vi "Teleop.vi"(10 "Match Info":T1={"Autonomous Elapsed Seconds"=0.0, "TeleOp Elapsed Seconds"=0.0, "Disabled Elapsed Seconds"=0.0, "Visited Autonomous"=FALSE, "Visited TeleOp"=FALSE, "Visited Disabled"=FALSE, "Autonomous Settings"={"Autonomous Style"=enum."Independent", "VI Refnum"=refnum}}, 11 "Call Context":T2) -> ()   [LabVIEW 2019]
doc: "This VI is called for each TeleOp packet received from the DS where the robot is not disabled. It is often used to read from the joysticks and update I/O or to update setpoints for timed control loops. It should complete and return within 20 milliseconds or it may miss DS packets."
uses:
  <vilib>/Rock Robotics/WPI/DriverStation/WPI_DriverStationDerivedRobotMode.ctl
  <vilib>/Rock Robotics/WPI/DriverStation/WPI_DriverStationMatch Info.ctl
  <vilib>/Rock Robotics/WPI/Utilities/WPI_GetSetVariantRefNum.vi
  <vilib>/Rock Robotics/Network Tables/NT Write Boolean Array.vi
  <vilib>/Rock Robotics/Network Tables/NT Write Numeric Array.vi
  <vilib>/Rock Robotics/Network Tables/NT Read Boolean.vi
  <vilib>/Rock Robotics/Network Tables/NT Read Number.vi
panel:
  out "Sample Slider 0":dbl(slide) scale=0.0..5.0
  out "Sample Boolean 1":bool
  out "Sample Boolean 0":bool
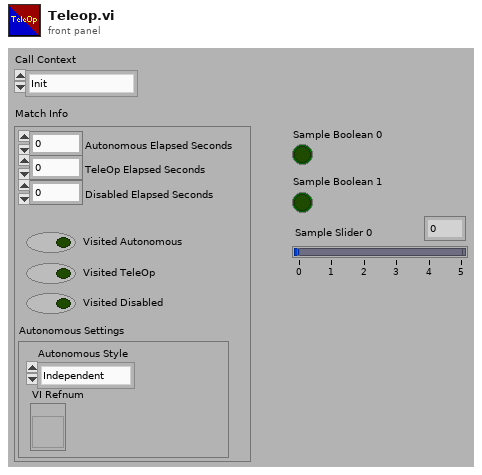
[diagram p1: front panel]
types:
  T1 = typedef "WPI_DriverStationMatch Info.ctl" = cluster{"Autonomous Elapsed Seconds":dbl, "TeleOp Elapsed Seconds":dbl, "Disabled Elapsed Seconds":dbl, "Visited Autonomous":bool, "Visited TeleOp":bool, "Visited Disabled":bool, "Autonomous Settings":cluster{"Autonomous Style":enum16{"Iterative", "Independent"}, "VI Refnum":refnum<vi>}}
  T2 = typedef "WPI_DriverStationDerivedRobotMode.ctl" = enum16{"Init", "Execute", "Stop"}
  T3 = typedef "WPI_RobotDriveDevRef.ctl" = cluster{"DevStatus":errorcluster, "Motors[]":T4[], "Square Inputs":bool, "Max Output":dbl}
  T4 = typedef "WPI_MotorControlDeviceRef.ctl" = cluster{"DeviceStatus":errorcluster, "Type":T5, "PWM":cluster{"PWM Channel":T6, "DeadBand":T7}, "CAN":cluster{"Device Number":u8, "SetOutput VI Ref":variant, "GetOutput VI Ref":variant, "Enable VI Ref":variant, "Disable VI Ref":variant, "Data":variant}, "Invert":bool, "DIO PWM":cluster{"PWM \"Enable\" Channel":T6, "DIOChannel":T8, "PWM Rate":dbl}}
  T5 = typedef "WPI_MotorControlType.ctl" = enum16{"PWM", "CAN", "DIO PWM"}
  T6 = typedef "FPGA_DIOPWMChannel.ctl" = enum8{"PWM 0", "PWM 1", "PWM 2", "PWM 3", "PWM 4", "PWM 5", "PWM 6", "PWM 7", "PWM 8", "PWM 9", "PWM MXP 0", "PWM MXP 1", "PWM MXP 2", "PWM MXP 3", "PWM MXP 4", "PWM MXP 5", "PWM MXP 6", "PWM MXP 7", "PWM MXP 8", "PWM MXP 9", "Invalid"}
  T7 = typedef "WPI_PWMDeadband.ctl" = cluster{"Name":string, "maxPositivePwm":i32, "minPositivePwm":i32, "centerPwm":i32, "maxNegativePwm":i32, "minNegativePwm":i32, "angularRange":u16}
  T8 = typedef "FPGA_DIOChannel.ctl" = enum8{"DIO 0", "DIO 1", "DIO 2", "DIO 3", "DIO 4", "DIO 5", "DIO 6", "DIO 7", "DIO 8", "DIO 9", "DIO MXP 0", "DIO MXP 1", "DIO MXP 2", "DIO MXP 3", "DIO MXP 4", "DIO MXP 5", "DIO MXP 6", "DIO MXP 7", "DIO MXP 8", "DIO MXP 9", "DIO MXP 10", "DIO MXP 11", "DIO MXP 12", "DIO MXP 13", "DIO MXP 14", "DIO MXP 15", "SPI Port CS1", "SPI Port CS2", "SPI Port CS3", "SPI Port MISO", "SPI Port MOSI", "Invalid"}
  T9 = typedef "WPI_JoystickDevRef.ctl" = cluster{"Device":T10}
  T10 = typedef "WPI_JoystickDeviceEnum.ctl" = enum16{"USB 0", "USB 1", "USB 2", "USB 3", "USB 4", "USB 5"}
  T11 = typedef "WPI_DigitalOutputDevRef.ctl" = cluster{"DIO Channel":T8, "DevStatus":errorcluster}
  T12 = typedef "WPI_AnalogChannelDevRef.ctl" = cluster{"DevStatus":errorcluster, "Analog Channel":T13}
  T13 = typedef "FPGA_AIChannel.ctl" = enum8{"AI 0", "AI 1", "AI 2", "AI 3", "AI MXP 0", "AI MXP 1", "AI MXP 2", "AI MXP 3", "Invalid"}
  T14 = typedef "WPI_GyroDevRef.ctl" = cluster{"DevStatus":errorcluster, "Analog Channel":T13, "Gain (VoltsPerDegree/Second)":dbl, "Gyro Type":enum16{"Analog", "XRS450"}, "Handle":i32, "SPI Bus":T15, "Device Found":bool, "Sample Rate":dbl, "Calibrate On Open":bool, "Offset":dbl}
  T15 = typedef "spi_bus.ctl" = enum16{"SPI On-Board, CS0", "SPI On-Board, CS1", "SPI On-Board, CS2", "SPI On-Board, CS3", "SPI MXP", "Invalid"}
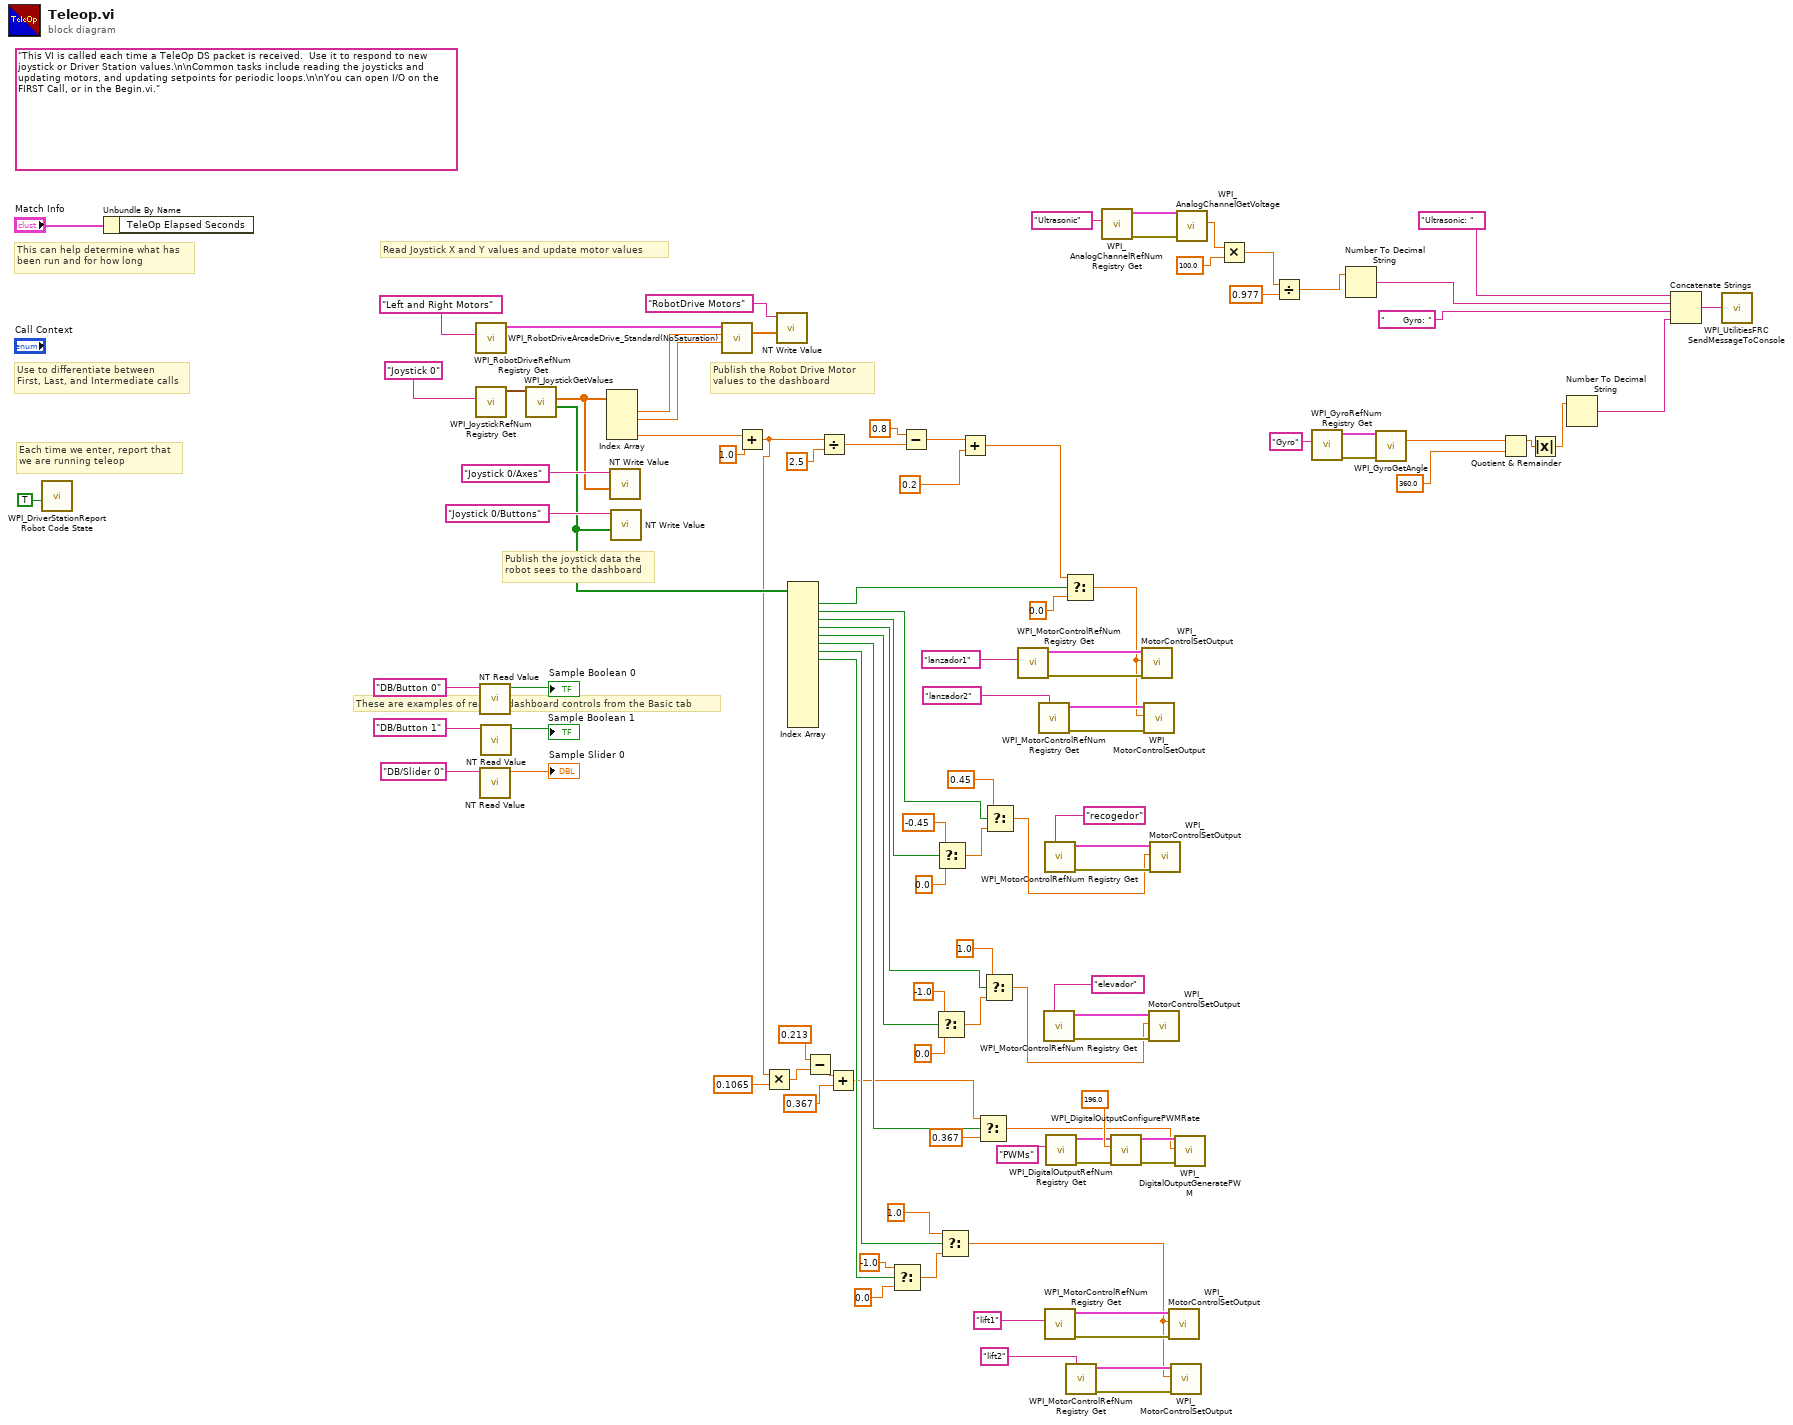
[diagram p0: block diagram]
diagram:
  (unwired) "This VI is called each time a TeleOp DS packet is received.  Use it to respond to new joystick or Driver Station values.\n\nCommon tasks include reading the joysticks and updating motors, and updating setpoints for periodic loops.\n\nYou can open I/O on the FIRST Call, or in the Begin.vi."
  # "These are examples of reading dashboard controls from the Basic tab"
  # "Publish the Robot Drive Motor\nvalues to the dashboard"
  # "Publish the joystick data the\nrobot sees to the dashboard"
  # "Each time we enter, report that\nwe are running teleop"
  # "Use to differentiate between\nFirst, Last, and Intermediate calls"
  # "This can help determine what has\nbeen run and for how long"
  # "Read Joystick X and Y values and update motor values"
  n1 = call <vilib>:"WPI_DriverStationReport Robot Code State.vi"("TeleOp"=TRUE ("Autonomous")) -> ()  [unwired: 10 in, 1 out]
  n2 = Unbundle By Name("Match Info") -> ()  [unwired: 1 out]
  n3 = call <vilib>:"WPI_RobotDriveRefNum Registry Get.vi"("refnum name"="Left and Right Motors") -> ("RobotDriveDevRef"=w103:T3)  [unwired: 1 in, 9 out]
  n4 = call <vilib>:"WPI_JoystickRefNum Registry Get.vi"("refnum name"="Joystick 0") -> ("JoystickDevRef"=w100:T9)  [unwired: 1 in, 9 out]
  n5 = call-poly <vilib>:"NT Read Value.vi"("Name"="DB/Button 0" ("refnum name")) -> ("Boolean"=→"Sample Boolean 0":bool)  [unwired: 9 in, 1 out]
  n6 = call-poly <vilib>:"NT Read Value.vi"("Name"="DB/Slider 0" ("refnum name")) -> ("Numeric"=→"Sample Slider 0":dbl)  [unwired: 9 in, 1 out]
  n7 = call-poly <vilib>:"NT Read Value.vi"("Name"="DB/Button 1" ("refnum name")) -> ("Boolean"=→"Sample Boolean 1":bool)  [unwired: 9 in, 1 out]
  n8 = call <vilib>:"WPI_JoystickGetValues.vi"("JoystickDevRef"=w100) -> ("Buttons"=w86:bool[], "Axes"=w95:dbl[])  [unwired: 6 in, 3 out]
  n9 = Index Array(array=w95) -> (element #1=w102:dbl, element #2=w98:dbl, element #4=w33:dbl)  [unwired: 4 in, 1 out]
  n10 = call-poly <vilib>:"NT Write Value.vi"("Numeric Array"=w95, "Name"="Joystick 0/Axes") -> ()  [unwired: 9 in, 1 out]
  n11 = call-poly <vilib>:"NT Write Value.vi"("Boolean Array"=w86, "Name"="Joystick 0/Buttons") -> ()  [unwired: 9 in, 1 out]
  n12 = call <vilib>:"WPI_RobotDriveArcadeDrive_Standard(NoSaturation).vi"("Y axis value"=w98, "X axis value"=w102, "RobotDriveDevRef"=w103) -> ("Motor Values"=w88:dbl[])  [unwired: 1 in, 7 out]
  n13 = Add(x=w33, y=1.0) -> (x+y=w11:dbl)
  n14 = Multiply(x=w11, y=0.1065) -> (x*y=w9:dbl)
  n15 = call-poly <vilib>:"NT Write Value.vi"("Numeric Array"=w88, "Name"="RobotDrive Motors") -> ()  [unwired: 9 in, 1 out]
  n16 = Index Array(array=w86) -> (element #1=w75:bool, element #2=w59:bool, element #3=w56:bool, element #4=w45:bool, element #5=w44:bool, element #6=w43:bool, element #7=w17:bool, element #8=w16:bool)  [unwired: 16 in, 8 out]
  n17 = Subtract(x=0.213, y=w9) -> (x-y=w7:dbl)
  n18 = Divide(x=w11, y=2.5) -> (x/y=w29:dbl)
  n19 = Add(x=w7, y=0.367) -> (x+y=w5:dbl)
  n20 = Select(t=-1.0, s=w16, f=0.0) -> (s? t:f=w18:dbl)
  n21 = Subtract(x=0.8, y=w29) -> (x-y=w28:dbl)
  n22 = Select(t=-1.0, s=w44, f=0.0 ("t")) -> (s? t:f=w48:dbl)
  n23 = Select(t=-0.45, s=w56, f=0.0 ("t")) -> (s? t:f=w57:dbl)
  n24 = Select(t=1.0, s=w17, f=w18) -> (s? t:f=w12:dbl)
  n25 = Add(x=w28, y=0.2) -> (x+y=w26:dbl)
  n26 = Select(t=w5, s=w43, f=0.367) -> (s? t:f=w13:dbl)
  n27 = Select(t=1.0, s=w45, f=w48) -> (s? t:f=w50:dbl)
  n28 = Select(t=0.45, s=w59, f=w57) -> (s? t:f=w60:dbl)
  n29 = call <vilib>:"WPI_MotorControlRefNum Registry Get.vi"("refnum name"="lanzador1") -> ("error out"=w83:errorcluster, "MotorControlDevRef"=w84:T4)  [unwired: 9 in]
  n30 = call <vilib>:"WPI_MotorControlRefNum Registry Get.vi"("refnum name"="lanzador2") -> ("error out"=w80:errorcluster, "MotorControlDevRef"=w81:T4)  [unwired: 9 in]
  n31 = call <vilib>:"WPI_MotorControlRefNum Registry Get.vi"("refnum name"="elevador") -> ("error out"=w52:errorcluster, "MotorControlDevRef"=w53:T4)  [unwired: 9 in]
  n32 = call <vilib>:"WPI_MotorControlRefNum Registry Get.vi"("refnum name"="recogedor") -> ("error out"=w77:errorcluster, "MotorControlDevRef"=w78:T4)  [unwired: 9 in]
  n33 = call <vilib>:"WPI_MotorControlRefNum Registry Get.vi"("refnum name"="lift1") -> ("error out"=w41:errorcluster, "MotorControlDevRef"=w42:T4)  [unwired: 9 in]
  n34 = call <vilib>:"WPI_DigitalOutputRefNum Registry Get.vi"("refnum name"="PWMs") -> ("error out"=w22:errorcluster, "DigitalOutputDevRef"=w23:T11)  [unwired: 9 in]
  n35 = Select(t=w26, s=w75, f=0.0) -> (s? t:f=w25:dbl)
  n36 = call <vilib>:"WPI_MotorControlRefNum Registry Get.vi"("refnum name"="lift2") -> ("error out"=w37:errorcluster, "MotorControlDevRef"=w38:T4)  [unwired: 9 in]
  n37 = call <vilib>:"WPI_AnalogChannelRefNum Registry Get.vi"("refnum name"="Ultrasonic") -> ("error out"=w73:errorcluster, "AIDeviceRef"=w74:T12)  [unwired: 9 in]
  n38 = call <vilib>:"WPI_DigitalOutputConfigurePWMRate.vi"("error in (no error)"=w22, "PWM Rate (Hz)"=sgl 196.0) -> ("error out"=w21:errorcluster)  [unwired: 8 in, 1 out]
  n39 = call <vilib>:"WPI_MotorControlSetOutput.vi"("error in (no error)"=w83, "Output"=w25, "MotorControlDevRef"=w84) -> ()  [unwired: 6 in, 3 out]
  n40 = call <vilib>:"WPI_MotorControlSetOutput.vi"("error in (no error)"=w80, "Output"=w25, "MotorControlDevRef"=w81) -> ()  [unwired: 6 in, 3 out]
  n41 = call <vilib>:"WPI_MotorControlSetOutput.vi"("error in (no error)"=w52, "Output"=w50, "MotorControlDevRef"=w53) -> ()  [unwired: 6 in, 3 out]
  n42 = call <vilib>:"WPI_MotorControlSetOutput.vi"("error in (no error)"=w77, "Output"=w60, "MotorControlDevRef"=w78) -> ()  [unwired: 6 in, 3 out]
  n43 = call <vilib>:"WPI_MotorControlSetOutput.vi"("error in (no error)"=w41, "Output"=w12, "MotorControlDevRef"=w42) -> ()  [unwired: 6 in, 3 out]
  n44 = call <vilib>:"WPI_MotorControlSetOutput.vi"("error in (no error)"=w37, "Output"=w12, "MotorControlDevRef"=w38) -> ()  [unwired: 6 in, 3 out]
  n45 = call <vilib>:"WPI_DigitalOutputGeneratePWM.vi"("error in (no error)"=w21, "PWM Duty Cycle"=w13, "DigitalOutputDevRef"=w23) -> ()  [unwired: 7 in, 2 out]
  n46 = call <vilib>:"WPI_AnalogChannelGetVoltage.vi"("error in (no error)"=w73, "AIDeviceRef"=w74) -> ("Voltage"=w71:dbl)  [unwired: 7 in, 2 out]
  n47 = Multiply(x=w71, y=100.0) -> (x*y=w69:dbl)
  n48 = Divide(x=w69, y=0.977) -> (x/y=w67:dbl)
  n49 = call <vilib>:"WPI_GyroRefNum Registry Get.vi"("refnum name"="Gyro") -> ("error out"=w63:errorcluster, "GyroDevRef"=w64:T14)  [unwired: 9 in]
  n50 = Number To Decimal String(number=w67) -> (decimal integer string=w65:string)  [unwired: 1 in]
  n51 = call <vilib>:"WPI_GyroGetAngle.vi"("error in"=w63, "GyroDevRef"=w64) -> ("Angle"=w4:dbl)  [unwired: 5 in, 4 out]
  n52 = Quotient & Remainder(x=w4, y=360.0) -> (x-y*floor(x/y)=w2:dbl)  [unwired: 1 out]
  n53 = Absolute Value(x=w2) -> (abs(x)=w1:dbl)
  n54 = Number To Decimal String(number=w1) -> (decimal integer string=w34:string)  [unwired: 1 in]
  n55 = Concatenate Strings("Ultrasonic: " ("string"), w65, "      Gyro: " ("string"), w34) -> (w61:string)
  n56 = call <vilib>:"WPI_UtilitiesFRC SendMessageToConsole.vi"("Message"=w61) -> ()  [unwired: 14 in, 1 out]
